vi "Gas Line Names.vi"() -> (1 "Gas line Names":string[](array[string]))   [LabVIEW 2022 SP3]
uses:
  Anemometry/Anemometry Sub Vis/Controls/GMU Gas Line Name.ctl
panel:
  in  "Gas Line Name":T1
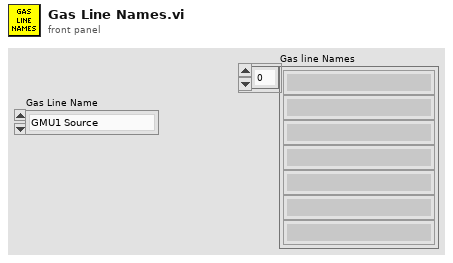
[diagram p1: front panel]
types:
  T1 = typedef "GMU Gas Line Name.ctl" = enum16{"GMU1 Source", "GMU2 Source", "GMU2 Calib", "CPP GRC-A", "CPP GRC-B"}
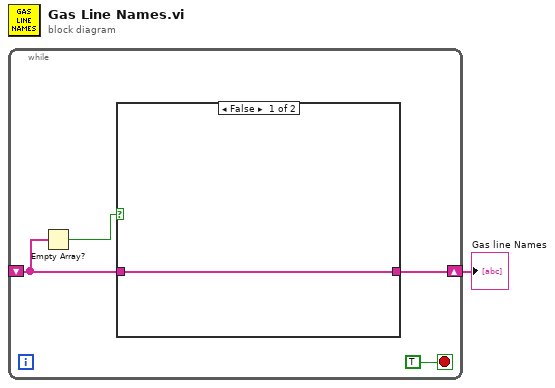
[diagram p0: block diagram]
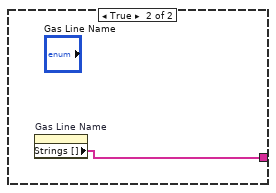
[diagram p2: hidden frame]
diagram:
  n1 = while {
    shift-right: [w3] -> w1
    shift-left: _ -> [w2]
    stop <- TRUE stop-if-true
    n2 = Empty Array?(array=w2) -> (empty?=w4:bool)
    n3 = case shown="False" w4 {
      tunnel: [w6 w7] -> w3
      tunnel: w2 -> [w6 _]
      frame False {
      }
      frame True {
        n4 = property on="Gas Line Name" class="Enum (strict)"() -> ("Strings []"=w7:string[])  [unwired: 2 in, 2 out]
      }
    }
  }
  "Gas line Names" <- w1
